vi "PH_ImageCalibrator.reset Attributes.vi"(0 "i ref in":refnum<vi>, 5 "error in (no error)":errorcluster) -> (14 "i ref out":refnum<vi>, 19 "error out":errorcluster)   [LabVIEW 2014, in "PH_ImageCalibrator.lvlib"]
doc: "This VI resets the attributes in case of a selecting another cam or canceling the calibration procedure, e.g.."
uses:
  PH_ImageCalibrator.lvlib
  PH_Img_BaseClass/PH_Img_BaseClass.lvlib
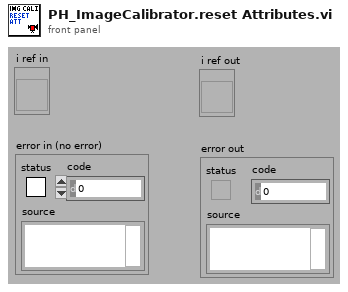
[diagram p1: front panel]
types:
  T1 = cluster{"Cam ID":string, "Gain":dbl, "Brightness":dbl, "Shutter":dbl, "Cam Error":bool, "Mode":i32}
  T2 = typedef "PH_ImageCalibrator.lvlib/PH_ImageCalibrator.i attribute.ctl" = cluster{"GUI Refs":cluster{"Available Cams":refnum<vi>, "OK":refnum<vi>, "Skip":refnum<vi>, "Repeat":refnum<vi>, "Cancel":refnum<vi>, "Length [mm]":refnum<vi>, "Energy [mJ]":refnum<vi>, "Dialog":refnum<vi>}, "Cam instances":string[], "Dark Pics":cluster{"#":i32, "BI taken":bool}, "Lin Cali":cluster{"Distance [Pixel]":dbl, "Distance [mm]":dbl, "Lin Cali Factor [mm/Pixel]":dbl}, "Energy Cali":cluster{"Pixelsum":dbl, "Energy [mJ]":dbl, "Energy Cali factor [mJ/Pixelsum]":dbl, "Underground subtracted?":bool, "#":i32}, "Images":cluster{"Background":T3, "Energy":T3}}
  T3 = typedef "IMAQ Image.ctl" = refnum<image>
  T4 = typedef "PH_Img_BaseClass.lvlib/PH_Img_BaseClass.i attribute.ctl" = cluster{"GUI Refs":T5, "Timeout Image [ms]":i32, "Default Periodic Period [ms]":i32, "Camera":cluster{"Instancename":string, "Notifier":refnum<notifier>}, "Palette":T6, "Cam Settings":cluster{"Cam ID":string, "Gain":dbl, "Brightness":dbl, "Shutter":dbl, "Cam Info Failure":bool, "Mode":i32}}
  T5 = typedef "PH_Img_BaseClass.lvlib/PH_Img_BaseClass.GUI Refs.ctl" = cluster{"Timeout":refnum<vi>, "Image":refnum<vi>, "Palette":refnum<vi>, "Timeout Set":refnum<vi>}
  T6 = typedef "PH_Img_BaseClass.lvlib/PH_Img_BaseClass.Palette.ctl" = i32
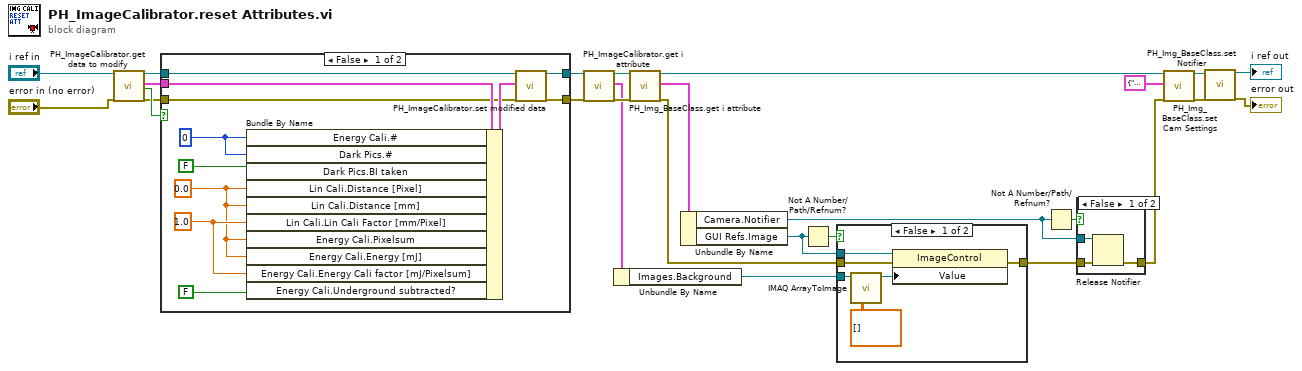
[diagram p0: block diagram]
diagram:
  n1 = call "PH_ImageCalibrator.get data to modify.vi"("i ref in"="i ref in", "error in (no error)"="error in (no error)") -> ("i ref out"=w20:refnum<vi>, "i attribute"=w22:T2, "timed out"=w23:bool, "error out"=w21:errorcluster)  [unwired: 14 in]
  n2 = case shown="False" w23 {
    tunnel: w20 -> [w37 w39]
    tunnel: w21 -> [w27 w38]
    tunnel: [w36 w39] -> w15
    tunnel: [w35 w38] -> w26
    tunnel: w22 -> [w29 _]
    frame False {
      w32 = 1.0 ("Energy Cali.Energy Cali factor [mJ/Pixelsum]")
      w31 = 0.0 ("Lin Cali.Distance [Pixel]")
      w28 = 0 ("Dark Pics.#")
      n3 = Bundle By Name(cluster=w29, "Energy Cali.#"=w28, "Dark Pics.#"=w28, "Dark Pics.BI taken"=FALSE, "Lin Cali.Distance [Pixel]"=w31, "Lin Cali.Distance [mm]"=w31, "Lin Cali.Lin Cali Factor [mm/Pixel]"=w32, "Energy Cali.Pixelsum"=w31, "Energy Cali.Energy [mJ]"=w31, "Energy Cali.Energy Cali factor [mJ/Pixelsum]"=w32, "Energy Cali.Underground subtracted?"=FALSE) -> (w34:T2)
      n4 = call "PH_ImageCalibrator.set modified data.vi"("i ref in"=w37, "i attribute"=w34, "error in (no error)"=w27) -> ("i ref out"=w36:refnum<vi>, "error out"=w35:errorcluster)  [unwired: 15 in]
    }
    frame True {
    }
  }
  n5 = call "PH_ImageCalibrator.get i attribute.vi"("i ref in"=w15, "error in (no error)"=w26) -> ("i ref out"=w14:refnum<vi>, "i attribute"=w13:T2, "error out"=w16:errorcluster)  [unwired: 15 in]
  n6 = Unbundle By Name(w13) -> ("Images.Background"=w2:T3)
  n7 = call "PH_Img_BaseClass.get i attribute.vi"("i ref in"=w14, "error in (no error)"=w16) -> ("i ref out"=w7:refnum<vi>, "i attribute"=w19:T4, "error out"=w12:errorcluster)  [unwired: 15 in]
  n8 = Unbundle By Name(w19) -> ("Camera.Notifier"=w11:refnum<notifier>, "GUI Refs.Image"=w17:refnum<vi>)
  n9 = Not A Number/Path/Refnum?(number/path/refnum=w17) -> (NaN/Path/Refnum?=w18:bool)
  n10 = case shown="False" w18 {
    tunnel: w17 -> [w45 _]
    tunnel: w12 -> [w44 w46]
    tunnel: [w43 w46] -> w9
    tunnel: w2 -> [w41 _]
    frame False {
      n11 = call "IMAQ ArrayToImage"("Image Pixels (Float)"=sgl[][] [], "Image"=w41) -> ("Image Out"=w42:T3)  [unwired: 8 in, 1 out]
      n12 = property class="ImageControl"(reference=w45, error in=w44, "Value"=w42) -> (error out=w43:errorcluster)  [unwired: 1 out]
    }
    frame True {
    }
  }
  n13 = Not A Number/Path/Refnum?(number/path/refnum=w11) -> (NaN/Path/Refnum?=w10:bool)
  n14 = case shown="False" w10 {
    tunnel: w11 -> [w49 _]
    tunnel: w9 -> [w48 w50]
    tunnel: [w47 w50] -> w3
    frame False {
      n15 = Release Notifier(notifier=w49, error in (no error)=w48) -> (error out=w47:errorcluster)  [unwired: 1 in, 2 out]
    }
    frame True {
    }
  }
  n16 = call "PH_Img_BaseClass.set Cam Settings.vi"("i ref in"=w7, "Cam Settings"=T1 {"Cam ID"="N/A", "Gain"=nan, "Brightness"=nan, "Shutter"=nan, "Cam Error"=TRUE, "Mode"=-1}, "error in (no error)"=w3) -> ("i ref out"=w8:refnum<vi>, "error out"=w5:errorcluster)  [unwired: 15 in]
  n17 = call "PH_Img_BaseClass.set Notifier.vi"("i ref in"=w8, "error in"=w5) -> ("i ref out"=→"i ref out":refnum<vi>, "error out"=→"error out":errorcluster)  [unwired: 16 in]
